vi "Triangle Area.vi"(6 "y 3":dbl, 7 "x 1":dbl, 8 "y 2":dbl, 9 "y 1":dbl, 10 "x 3":dbl, 11 "x 2":dbl) -> (3 "area":dbl)   [LabVIEW 2020, in "NI_AAL_Geometry.lvlib"]
uses:
  <vilib>/Analysis/NI_AAL_Geometry.lvlib
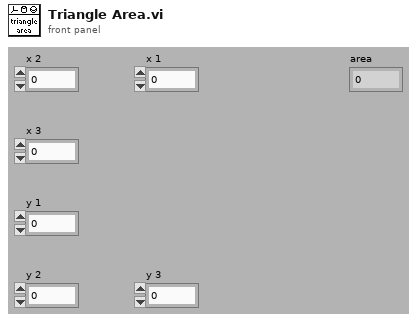
[diagram p1: front panel]
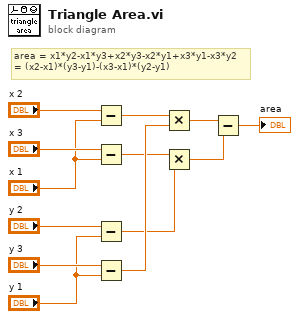
[diagram p0: block diagram]
diagram:
  # "area = x1*y2-x1*y3+x2*y3-x2*y1+x3*y1-x3*y2\n= (x2-x1)*(y3-y1)-(x3-x1)*(y2-y1)"
  n1 = Subtract(x="x 2", y="x 1") -> (x-y=w12:dbl)
  n2 = Subtract(x="x 3", y="x 1") -> (x-y=w6:dbl)
  n3 = Subtract(x="y 2", y="y 1") -> (x-y=w3:dbl)
  n4 = Subtract(x="y 3", y="y 1") -> (x-y=w10:dbl)
  n5 = Multiply(x=w12, y=w10) -> (x*y=w9:dbl)
  n6 = Multiply(x=w6, y=w3) -> (x*y=w5:dbl)
  n7 = Subtract(x=w9, y=w5) -> (x-y=→"area":dbl)
